vi "measureTOmT.vi"(5 "string":string, 11 "error in (no error)":errorcluster) -> (6 "Numeric":dbl, 8 "String":string, 15 "error out":errorcluster)   [LabVIEW 2014, in "FH 55.lvlib"]
uses:
  FH 55.lvlib
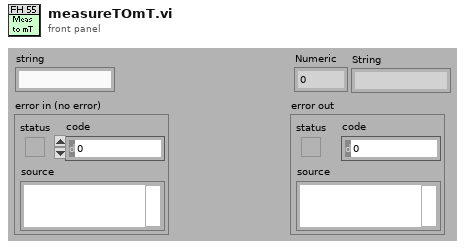
[diagram p1: front panel]
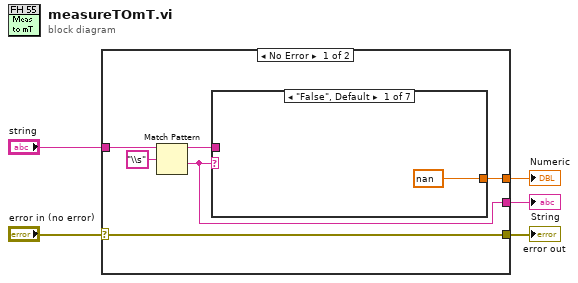
[diagram p0: block diagram]
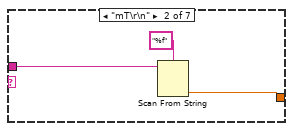
[diagram p2: hidden frame]
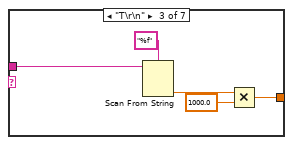
[diagram p3: hidden frame]
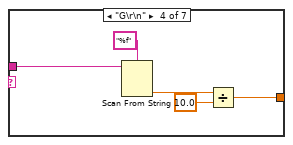
[diagram p4: hidden frame]
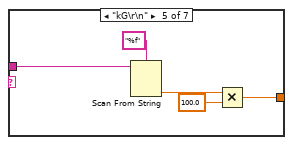
[diagram p5: hidden frame]
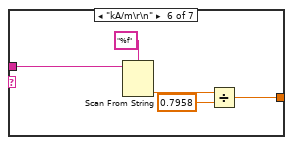
[diagram p6: hidden frame]
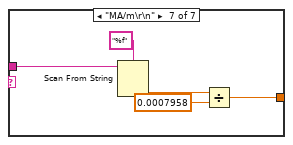
[diagram p7: hidden frame]
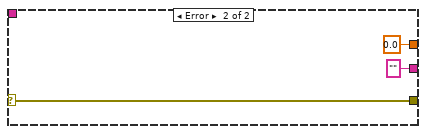
[diagram p8: hidden frame]
diagram:
  n1 = case shown="No Error" "error in (no error)" {
    selector: "error in (no error)" -> [w7 w43]
    tunnel: [w10 0.0] -> w5
    tunnel: "string" -> [w8 _]
    tunnel: [w7 w43] -> w2
    tunnel: [w6 "" ("string")] -> w1
    frame No Error {
      n2 = Match Pattern(string=w8, regular expression="\\s") -> (before substring=w9:string, after substring=w6:string)  [unwired: 1 in, 2 out]
      n3 = case shown="\"False\", Default" w6 {
        tunnel: [nan w14 w17 w22 w27 w32 w37] -> w10
        tunnel: w9 -> [_ w13 w16 w21 w26 w31 w36]
        frame "False", Default {
        }
        frame "mT\r\n" {
          n4 = Scan From String(format string="%f", input string=w13) -> (output 1=w14:dbl)  [unwired: 3 in, 3 out]
        }
        frame "T\r\n" {
          n5 = Scan From String(format string="%f", input string=w16) -> (output 1=w19:dbl)  [unwired: 3 in, 3 out]
          n6 = Multiply(x=w19, y=1000.0) -> (x*y=w17:dbl)
        }
        frame "G\r\n" {
          n7 = Scan From String(format string="%f", input string=w21) -> (output 1=w24:dbl)  [unwired: 3 in, 3 out]
          n8 = Divide(x=w24, y=10.0) -> (x/y=w22:dbl)
        }
        frame "kG\r\n" {
          n9 = Scan From String(format string="%f", input string=w26) -> (output 1=w29:dbl)  [unwired: 3 in, 3 out]
          n10 = Multiply(x=w29, y=100.0) -> (x*y=w27:dbl)
        }
        frame "kA/m\r\n" {
          n11 = Scan From String(format string="%f", input string=w31) -> (output 1=w34:dbl)  [unwired: 3 in, 3 out]
          n12 = Divide(x=w34, y=0.7958) -> (x/y=w32:dbl)
        }
        frame "MA/m\r\n" {
          n13 = Scan From String(format string="%f", input string=w36) -> (output 1=w39:dbl)  [unwired: 3 in, 3 out]
          n14 = Divide(x=w39, y=0.0007958) -> (x/y=w37:dbl)
        }
      }
    }
    frame Error {
    }
  }
  "Numeric" <- w5
  "error out" <- w2
  "String" <- w1
